vi "Self Event Alias.vi"(11 "Event in":refnum<class "Event.lvclass">) -> (2 "Self Event Alias":string)   [LabVIEW 2021, in "jettl.lvlib" / "Event.lvclass"]
uses:
  Event.lvclass
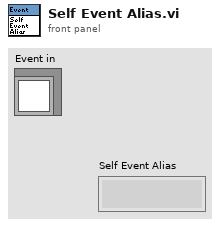
[diagram p1: front panel]
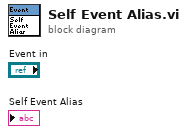
[diagram p0: block diagram]
diagram:
